vi "Config.vi"(8 "error in (no error)":errorcluster, 10 "size (10)":u32, 11 "dY_dX_Calculator in":refnum<class "delayValue.lvclass">) -> (0 "error out":errorcluster, 3 "dY_dX_Calculator out":refnum<class "delayValue.lvclass">)   [LabVIEW 2019, in "delayValue.lvclass"]
uses:
  delayValue.lvclass
  delayValue.lvclass/delayValue.ctl
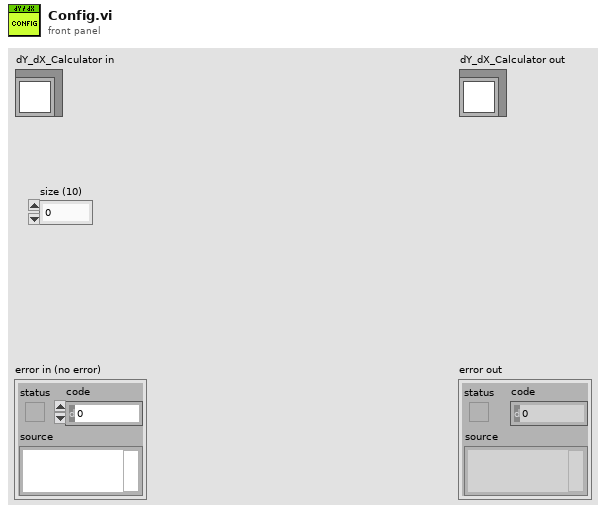
[diagram p1: front panel]
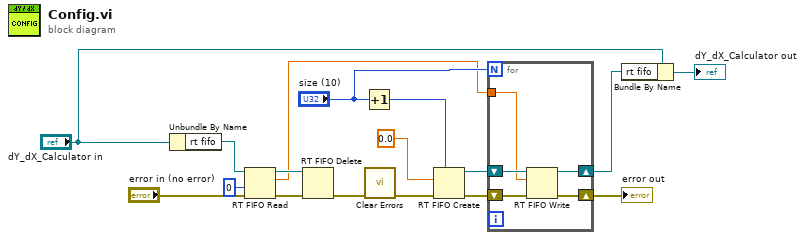
[diagram p0: block diagram]
diagram:
  n1 = Unbundle By Name("dY_dX_Calculator in") -> ("rt fifo"=w6:refnum<k33>)
  n2 = RT FIFO Read(0:w6, 2:0 ("timeout in ms (0)"), 3:"error in (no error)") -> (8:w3:refnum<k33>, 9:w2:dbl, 11:w4:errorcluster)  [unwired: 1 in, 2 out]
  n3 = RT FIFO Delete(0:w3, 3:w4) -> (11:w16:errorcluster)  [unwired: 1 in]
  n4 = Increment(x="size (10)") -> (x+1=w14:u32)
  n5 = call <vilib>:"Clear Errors.vi"("error in (no error)"=w16) -> ("error out"=w15:errorcluster)  [unwired: 5 in, 1 out]
  n6 = RT FIFO Create(1:0.0, 3:w15, 4:w14) -> (8:w13:refnum<k33>, 11:w12:errorcluster)  [unwired: 5 in, 1 out]
  n7 = for {
    N: "size (10)" -> [_]
    shift-right: [w21] -> w10
    shift-left: w13 -> [w22]
    shift-right: [w19] -> w9
    shift-left: w12 -> [w20]
    tunnel: w2 -> [w18]
    n8 = RT FIFO Write(0:w22, 1:w18, 3:w20) -> (8:w21:refnum<k33>, 11:w19:errorcluster)  [unwired: 2 in, 2 out]
  }
  "error out" <- w9
  n9 = Bundle By Name(cluster="dY_dX_Calculator in", "rt fifo"=w10) -> (→"dY_dX_Calculator out":refnum<class "delayValue.lvclass">)
